vi "timedependent_writing_reading_and_waveform_chart.vi"() -> ()   [LabVIEW 2019]
panel:
  out "String 2":string
  out "sıcaklık3_oku":dbl
  out "sıcaklık2_oku":dbl
  out "sıcaklık1_oku":dbl
  out "Waveform Chart 2":dbl[](graph)
  out "text":string
  out "subarray":dbl[](array[numeric])
  in  "stop 2":bool
  in  "Veri Oku":bool
  out "Döngü 2":i32
  out "String":string
  out "sıcaklık3":dbl
  out "sıcaklık2":dbl
  out "sıcaklık1":dbl
  in  "stop":bool
  out "Döngü":i32
  out "Waveform Chart":dbl[](graph)
  in  "file path":path
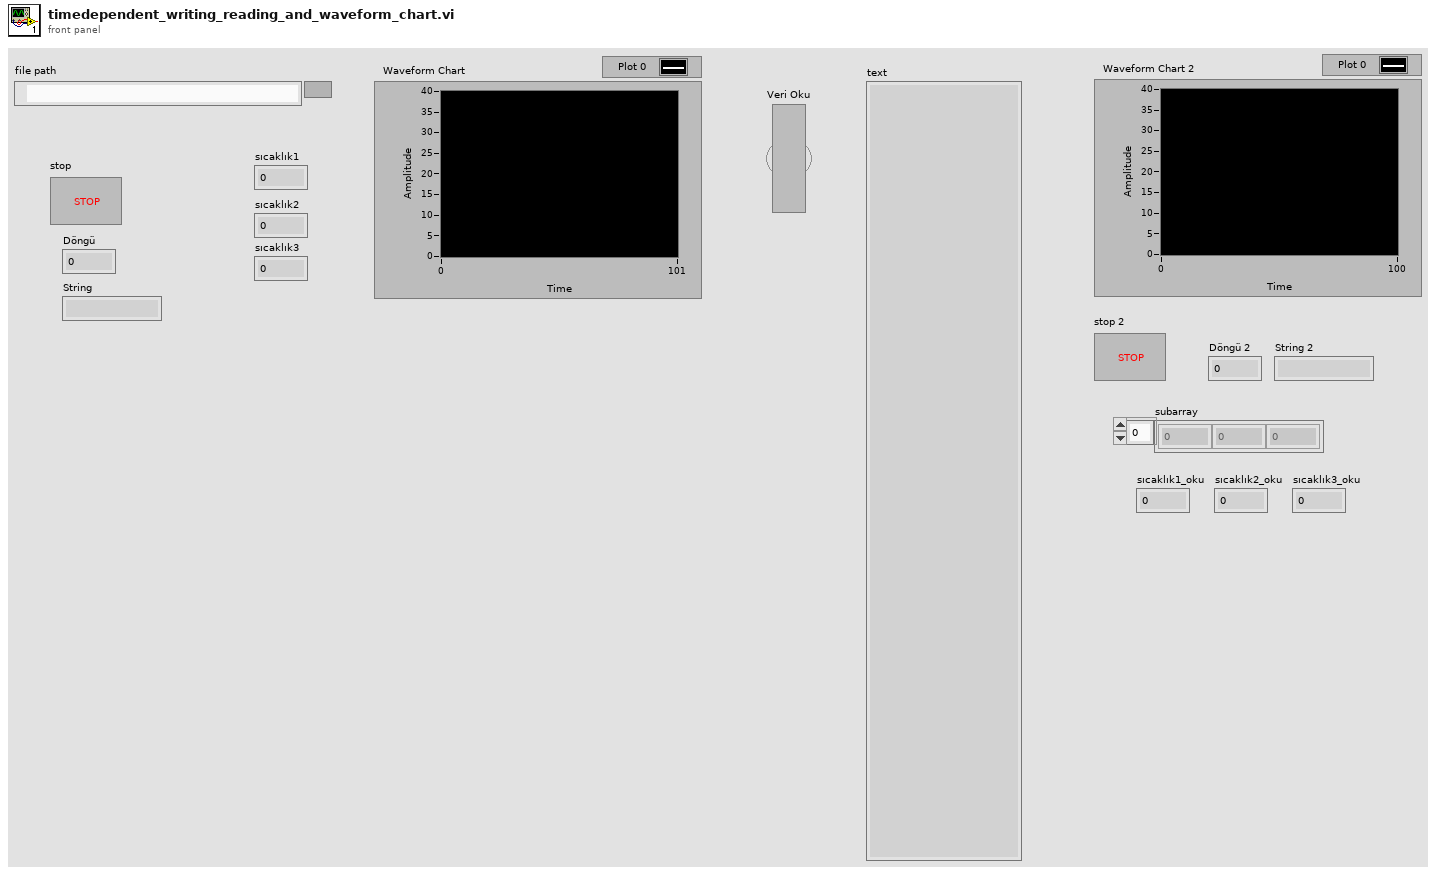
[diagram p1: front panel]
types:
  T1 = enum16{"open", "replace", "create", "open or create", "replace or create", "replace or create with confirmation"}
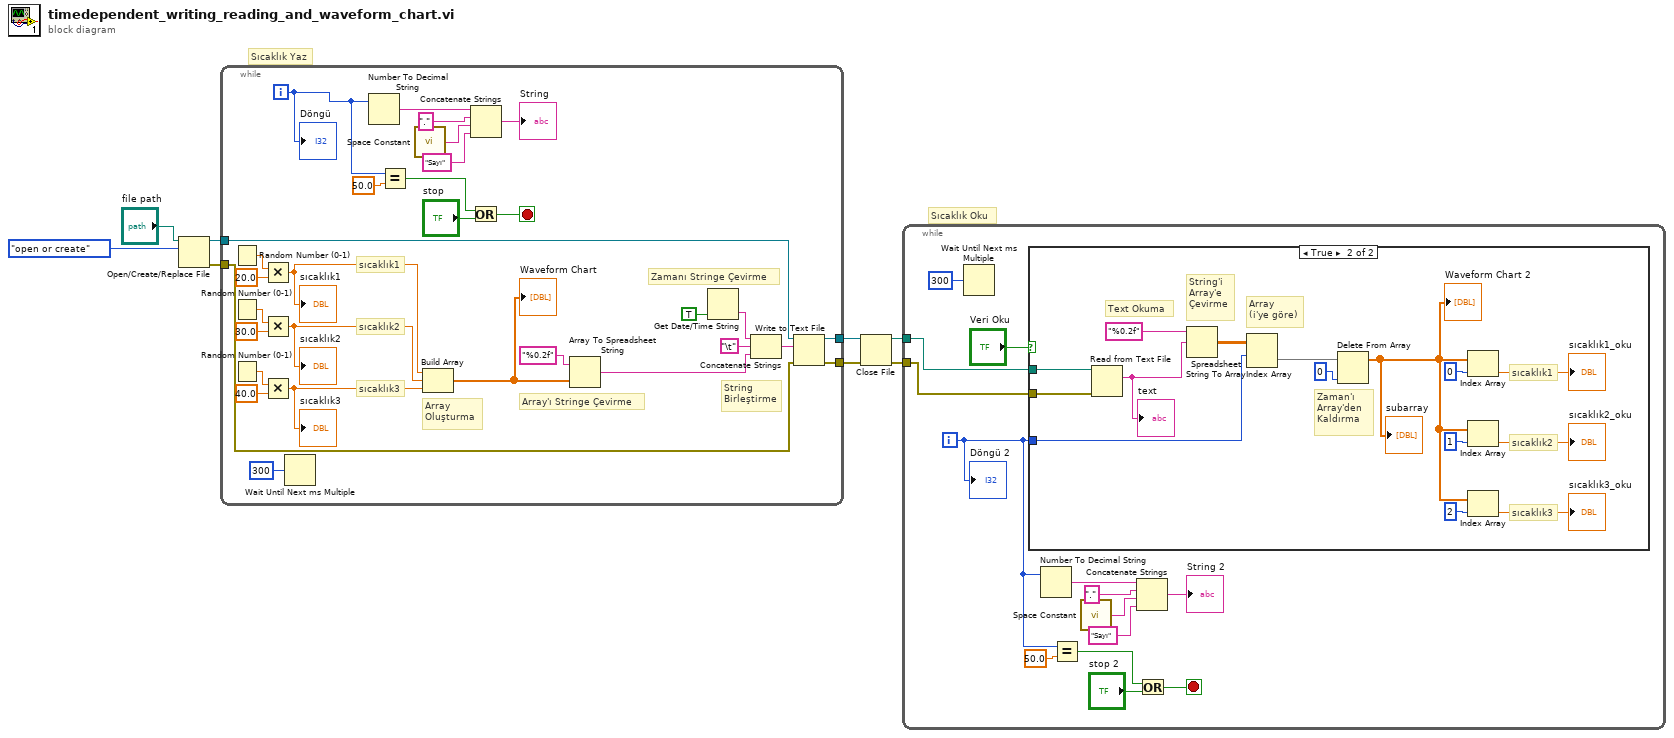
[diagram p0: block diagram]
diagram:
  # "Sıcaklık Oku"
  # "Sıcaklık Yaz"
  n1 = Open/Create/Replace File(file path (use dialog)="file path", operation (0:open)=T1."open or create") -> (refnum out=w6:refnum<file>, error out=w3:errorcluster)  [unwired: 4 in, 1 out]
  n2 = while {
    tunnel: w6 -> [w39]
    tunnel: [w38] -> w5
    tunnel: [w37] -> w4
    tunnel: w3 -> [w36]
    i -> [w14]
    stop <- w25 stop-if-true
    # "String \nBirleştirme"
    # "Array'ı Stringe Çevirme"
    # "Zamanı Stringe Çevirme"
    # "Array \nOluşturma"
    # "sıcaklık3"
    # "sıcaklık2"
    # "sıcaklık1"
    n3 = Random Number (0-1)() -> (number: 0 to 1=w35:dbl)
    n4 = Random Number (0-1)() -> (number: 0 to 1=w23:dbl)
    n5 = Random Number (0-1)() -> (number: 0 to 1=w21:dbl)
    n6 = Multiply(x=w35, y=20.0) -> (x*y=w18:dbl)
    "sıcaklık1" <- w18
    n7 = Multiply(x=w23, y=30.0) -> (x*y=w17:dbl)
    "sıcaklık2" <- w17
    n8 = Multiply(x=w21, y=40.0) -> (x*y=w16:dbl)
    "sıcaklık3" <- w16
    n9 = Wait Until Next ms Multiple(millisecond multiple=u32 300) -> ()  [unwired: 1 out]
    n10 = Number To Decimal String(number=w14) -> (decimal integer string=w9:string)  [unwired: 1 in]
    n11 = Equal?(x=w14, y=50.0) -> (x = y?=w24:bool)
    n12 = call <vilib>:"Space Constant.vi"() -> ("String"=w12:string)
    n13 = Build Array(w18, w17, w16) -> (w32:dbl[])
    "Waveform Chart" <- w32
    n14 = Concatenate Strings(w9, "." ("string"), w12, "Sayı" ("string")) -> (→"String":string)
    n15 = Or(x=w24, y="stop") -> (x .or. y?=w25:bool)
    n16 = Array To Spreadsheet String(array=w32, 3:"%0.2f" ("format string")) -> (spreadsheet string=w29:string)  [unwired: 1 in]
    n17 = Get Date/Time String(want seconds? (F)=TRUE) -> (time string=w31:string)  [unwired: 2 in, 1 out]
    n18 = Concatenate Strings(w31, "\t", w29) -> (w15:string)
    n19 = Write to Text File(file (use dialog)=w39, text=w15, error in=w36) -> (refnum out=w38:refnum<file>, error out=w37:errorcluster)  [unwired: 1 in, 1 out]
    "Döngü" <- w14
  }
  n20 = Close File(refnum=w5, error in=w4) -> (path=w2:path, error out=w1:errorcluster)
  n21 = while {
    tunnel: w2 -> [w51]
    tunnel: w1 -> [w50]
    i -> [w44]
    stop <- w45 stop-if-true
    n22 = Wait Until Next ms Multiple(millisecond multiple=u32 300) -> ()  [unwired: 1 out]
    n23 = case shown="True" "Veri Oku" {
      tunnel: w51 -> [_ w68]
      tunnel: w50 -> [_ w67]
      tunnel: w44 -> [_ w64]
      frame False {
      }
      frame True {
        # "String'i \nArray'e \nÇevirme"
        # "sıcaklık3"
        # "sıcaklık2"
        # "sıcaklık1"
        # "Zaman'ı Array'den Kaldırma"
        # "Array\n(i'ye göre)"
        # "Text Okuma"
        n24 = Read from Text File(file (use dialog)=w68, error in=w67) -> (text=w65:string)  [unwired: 2 in, 3 out]
        "text" <- w65
        n25 = Spreadsheet String To Array(format string="%0.2f", spreadsheet string=w65) -> (array=w63:dbl[][])  [unwired: 2 in]
        n26 = Index Array(array=w63, index (row)=w64) -> (element=w57:dbl[])  [unwired: 1 in]
        n27 = Delete From Array(array=w57, index=0) -> (array with subset deleted=w55:dbl[])  [unwired: 1 in, 1 out]
        "Waveform Chart 2" <- w55
        "subarray" <- w55
        n28 = Index Array(array=w55, index=0) -> (element=→"sıcaklık1_oku":dbl)
        n29 = Index Array(array=w55, index=1) -> (element=→"sıcaklık2_oku":dbl)
        n30 = Index Array(array=w55, index=2) -> (element=→"sıcaklık3_oku":dbl)
      }
    }
    n31 = Number To Decimal String(number=w44) -> (decimal integer string=w43:string)  [unwired: 1 in]
    n32 = Equal?(x=w44, y=50.0) -> (x = y?=w48:bool)
    n33 = call <vilib>:"Space Constant.vi"() -> ("String"=w41:string)
    n34 = Concatenate Strings(w43, "." ("string"), w41, "Sayı" ("string")) -> (→"String 2":string)
    n35 = Or(x=w48, y="stop 2") -> (x .or. y?=w45:bool)
    "Döngü 2" <- w44
  }
